vi "UHR-Fleezers Control (host) - 11.9b.vi"() -> ()   [LabVIEW 2014] (continued)
        n1560 = Add(x=w2217, y=w2214) -> (x+y=w2215:i64)
        n1561 = local write "Trap Pos. FB Offset Factor"(w2215) -> ()
        n1562 = xnode "Read/Write Control"("FPGA VI Reference In"=w2221, "error in"=w2220, "Trap Pos. FB Offset Factor"=w2215) -> ()  [unwired: 2 out]
      }
      event "Remove Offset to factor": Value Change {
        n1563 = event-data() -> ()  [unwired: 7 out]
        n1564 = local write "Remove Offset to factor"(FALSE ("Remove Action Offset")) -> ()
        n1565 = local read "Trap Pos. FB Mult Factor"() -> (w2233:i64)
        n1566 = local read "Trap Pos FB Action"() -> (w2231:i64)
        n1567 = local read "Trap Pos. FB Offset Factor"() -> (w2230:i64)
        n1568 = Multiply(x=w2233, y=w2231) -> (x*y=w2232:i64)
        n1569 = local read "Trap Pos. FB Mult Factor"() -> (w2229:i64)
        n1570 = Add(x=w2232, y=w2230) -> (x+y=w2224:i64)
        n1571 = Multiply(x=32768, y="factor") -> (x*y=w2227:dbl)
        n1572 = Multiply(x=w2227, y=w2229) -> (x*y=w2228:dbl)
        n1573 = Subtract(x=w2224, y=w2228) -> (x-y=w2222:dbl)
        n1574 = To Quad Integer(1:w2222) -> (0:w2223:i64)
        n1575 = xnode "Read/Write Control"("FPGA VI Reference In"=w2236, "error in"=w2235, "Trap Pos. FB Offset Factor"=w2223) -> ()  [unwired: 2 out]
        n1576 = local write "Trap Pos. FB Offset Factor"(w2223) -> ()
      }
      event "Trap Pos. FB Range", "Trap Pos. FB Gains", "Trap Pos. FB Mult Factor", "Trap Pos. FB Offset Factor", "Trap Pos FB Negate Action", "Trap Pos FB Monitor\nT1 or T2", "Differential FB?", "Negate Diff?": Value Change {
        n1577 = event-data() -> ()  [unwired: 7 out]
        n1578 = local read "Negate Diff?"() -> (w2237:bool)
        n1579 = xnode "Read/Write Control"("FPGA VI Reference In"=w2247, "error in"=w2246, "Trap Pos. FB Range"="Trap Pos. FB Range", "Trap Pos. FB Gains"="Trap Pos. FB Gains", "Trap Pos. FB Mult Factor"="Trap Pos. FB Mult Factor", "Trap Pos. FB Offset Factor"="Trap Pos. FB Offset Factor", "Trap Pos FB Negate Action"="Trap Pos FB Negate Action", "Trap Pos FB Monitor T1 or T2"="Trap Pos FB Monitor\nT1 or T2", "AI1 X Scale"="Trap Pos. AI1 X Pre-scale", "Negate Diff?"=w2237, "Diff FB Measurement?"="Differential FB?") -> ()  [unwired: 2 out]
      }
      event "Trap Pos FB SP", "Trap Pos FB SP 2", "Use SP 2": Value Change {
        n1580 = event-data() -> ()  [unwired: 7 out]
        n1581 = Select(t="Trap Pos FB SP 2", s="Use SP 2", f="Trap Pos FB SP") -> (s? t:f=w2248:fxp<+/-,16,1>)
        n1582 = xnode "Read/Write Control"("FPGA VI Reference In"=w2253, "error in"=w2252, "Trap Pos. FB SP"=w2248) -> ()  [unwired: 2 out]
      }
      event "Offset SP2 from SP1": Value Change {
        n1583 = event-data() -> ()  [unwired: 7 out]
        n1584 = local read "Trap Pos FB SP"() -> (w2256:fxp<+/-,16,1>)
        n1585 = Add(x=w2256, y="SP2 Offset") -> (x+y=w2254:fxp<+/-,16,1>)
        n1586 = property on="Trap Pos FB SP 2" class="DigNum (strict)"("Val(Sgnl)"=w2254) -> ()  [unwired: 2 in, 2 out]
        n1587 = local write "Offset SP2 from SP1"(FALSE ("Offset SP2 from SP1")) -> ()
      }
      event "Set Reading to\nSetpoint": Value Change {
        # "This is the actual PID input signal"
        n1588 = event-data() -> ()  [unwired: 7 out]
        n1589 = local write "Set Reading to\nSetpoint"(FALSE ("Set SP to Reading")) -> ()
        n1590 = xnode "Read/Write Control"("FPGA VI Reference In"=w2262, "error in"=w2261) -> ("FPGA VI Reference Out"=w2260:T19, "error out"=w2259:errorcluster, "Trap Pos FB Int-Norm Signal"=w2258:fxp<+/-,16,1>)
        n1591 = local read "Differential FB?"() -> (w2263:bool)
        n1592 = case shown="False" w2263 {
          tunnel: [w2268 w2275] -> w2265
          tunnel: w2258 -> [w2266 w2275]
          frame False {
            n1593 = local read "Trap Pos FB Monitor\nT1 or T2"() -> (w2271:bool)
            n1594 = local read "Trap X AI1 (DMA)"() -> (w2274:T13)
            n1595 = Unbundle By Name(w2274) -> ("Set 1"=w2273:fxp<+/-,16,1>, "Set 2"=w2272:fxp<+/-,16,1>)
            n1596 = Select(t=w2273, s=w2271, f=w2272) -> (s? t:f=w2270:fxp<+/-,16,1>)
            n1597 = Not(x="Set SP Using...") -> (.not. x?=w2267:bool)
            n1598 = Select(t=w2266, s=w2267, f=w2270) -> (s? t:f=w2268:fxp<+/-,16,1>)
          }
          frame True {
          }
        }
        n1599 = xnode "Read/Write Control"("FPGA VI Reference In"=w2260, "error in"=w2259, "Trap Pos. FB SP"=w2265) -> ()  [unwired: 2 out]
        n1600 = local write "Trap Pos FB SP"(w2265) -> ()
      }
      event "Trap Pos. FB Out Scale 2^n": Value Change {
        n1601 = event-data() -> ()  [unwired: 7 out]
        n1602 = Scale By Power Of 2(n="Trap Pos. FB Out Scale 2^n", x=ext 1.0) -> (x*2^n=w2276:ext)
        n1603 = property on="Trap Pos. FB Mult Factor" class="DigNum (strict)"("Val(Sgnl)"=w2276) -> ()  [unwired: 2 in, 2 out]
      }
      event "Trap Pos FB Int Count": Value Change {
        n1604 = event-data() -> ()  [unwired: 7 out]
        n1605 = xnode "Read/Write Control"("FPGA VI Reference In"=w2281, "error in"=w2280, "Trap Pos FB Int Count"="Trap Pos FB Int Count") -> ()  [unwired: 2 out]
      }
      event "Trap pos": Value Change {
        n1606 = event-data() -> ()  [unwired: 7 out]
        n1607 = case shown="True" "Trap pos" {
          frame False {
            n1608 = property on="Trap Delta Graph" class="WFGraph (strict)"("Visible"=TRUE) -> ()  [unwired: 2 in, 2 out]
            n1609 = property on="Saved trap pos" class="WFGraph (strict)"("Visible"=FALSE) -> ()  [unwired: 2 in, 2 out]
          }
          frame True {
            n1610 = property on="Saved trap pos" class="WFGraph (strict)"("Visible"=TRUE) -> ()  [unwired: 2 in, 2 out]
            n1611 = property on="Trap Delta Graph" class="WFGraph (strict)"("Visible"=FALSE) -> ()  [unwired: 2 in, 2 out]
          }
        }
      }
      event "Save user params": Value Change {
        n1612 = event-data() -> ()  [unwired: 7 out]
        n1613 = local write "Save user params"(FALSE ("Save user\nparams")) -> ()
        n1614 = call "save control values.vi"("User"="User") -> ()  [unwired: 8 in, 1 out]
        n1615 = local read "Messages"() -> (w2293:string)
        n1616 = Concatenate Strings("User: ", "User", "\r", "Parameters saved.") -> (w2288:string)
        n1617 = call "Update messages.vi"("Message to add"=w2288, "Old message string"=w2293) -> ("New message string"=w2287:string)
        n1618 = local write "Messages"(w2287) -> ()
      }
      event "Load user params": Value Change {
        n1619 = event-data() -> ()  [unwired: 7 out]
        n1620 = local write "Load user params"(FALSE ("Read user\nparams")) -> ()
        n1621 = flat-sequence {
          tunnel: [w2325] -> w2313
          tunnel: [w2324] -> w2311
          tunnel: [w2323] -> w2309
          tunnel: [w2322] -> w2307
          tunnel: [w2321] -> w2305
          tunnel: [w2320] -> w2303
          tunnel: [w2319] -> w2301
          tunnel: [w2318] -> w2299
          tunnel: [w2317] -> w2297
          tunnel: [w2316] -> w2295
          tunnel: [w2335] -> w2314
          tunnel: w2313 -> [w2335]
          tunnel: [w2334] -> w2312
          tunnel: w2311 -> [w2334]
          tunnel: [w2333] -> w2310
          tunnel: w2309 -> [w2333]
          tunnel: [w2332] -> w2308
          tunnel: w2307 -> [w2332]
          tunnel: [w2331] -> w2306
          tunnel: w2305 -> [w2331]
          tunnel: [w2330] -> w2304
          tunnel: w2303 -> [w2330]
          tunnel: [w2329] -> w2302
          tunnel: w2301 -> [w2329]
          tunnel: [w2328] -> w2300
          tunnel: w2299 -> [w2328]
          tunnel: [w2327] -> w2298
          tunnel: w2297 -> [w2327]
          tunnel: [w2326] -> w2296
          tunnel: w2295 -> [w2326]
          tunnel: w2314 -> [w2352]
          tunnel: w2312 -> [w2351]
          tunnel: w2310 -> [w2350]
          tunnel: w2308 -> [w2349]
          tunnel: w2306 -> [w2348]
          tunnel: w2304 -> [w2347]
          tunnel: w2302 -> [w2346]
          tunnel: w2300 -> [w2345]
          tunnel: w2298 -> [w2344]
          tunnel: w2296 -> [w2343]
          frame #0 {
            # "Make exceptions.\nThese will not be\nloaded."
            n1622 = local read "Sample Channel\nFlow"() -> (w2320:bool)
            n1623 = local read "Green ON/Interlacing"() -> (w2321:bool)
            n1624 = local read "Trap 1 (ON/OFF)"() -> (w2325:bool)
            n1625 = local read "Trap 2 (ON/OFF)"() -> (w2324:bool)
            n1626 = local read "Trap Pos. FB ON"() -> (w2316:bool)
            n1627 = local read "Inject Pump 1"() -> (w2319:bool)
            n1628 = local read "Inject Pump 3"() -> (w2318:bool)
            n1629 = local read "Trap D (MHz)"() -> (w2317:dbl)
            n1630 = local read "Index"() -> (w2322:dbl)
            n1631 = local read "Fish"() -> (w2323:bool)
          }
          frame #1 {
            n1632 = local read "User"() -> (w2336:string)
            n1633 = call "retrieve control values.vi"("User"=w2336) -> ()  [unwired: 10 in, 1 out]
            n1634 = local read "Messages"() -> (w2342:string)
            n1635 = Concatenate Strings("User: ", w2336, "\r", "Parameters loaded.") -> (w2337:string)
            n1636 = call "Update messages.vi"("Message to add"=w2337, "Old message string"=w2342) -> ("New message string"=w2341:string)
            n1637 = local write "Messages"(w2341) -> ()
          }
          frame #2 {
            n1638 = local write "Sample Channel\nFlow"(w2347) -> ()
            n1639 = local write "Green ON/Interlacing"(w2348) -> ()
            n1640 = local write "Trap 1 (ON/OFF)"(w2352) -> ()
            n1641 = local write "Trap 2 (ON/OFF)"(w2351) -> ()
            n1642 = local write "Inject Pump 1"(w2346) -> ()
            n1643 = local write "Trap Pos. FB ON"(w2343) -> ()
            n1644 = local write "Inject Pump 3"(w2345) -> ()
            n1645 = local write "Trap D (MHz)"(w2344) -> ()
            n1646 = local write "Index"(w2349) -> ()
            n1647 = local write "Fish"(w2350) -> ()
          }
        }
      }
      event "Abort wiggle": Value Change {
        n1648 = event-data() -> ()  [unwired: 7 out]
        n1649 = flat-sequence {
          tunnel: w2356 -> [w2360]
          tunnel: w2355 -> [w2359]
          tunnel: [w2358] -> w2353
          tunnel: [w2362] -> w2354
          tunnel: w2353 -> [w2362]
          frame #0 {
            n1650 = xnode "Read/Write Control"("FPGA VI Reference In"=w2360, "error in"=w2359, "Abort wiggle 1"="Abort wiggle", "Abort wiggle 2"="Abort wiggle") -> ("error out"=w2358:errorcluster)  [unwired: 1 out]
          }
          frame #1 {
            n1651 = local write "Abort wiggle"(FALSE ("Abort wiggle")) -> ()
          }
        }
      }
    }
    "error out 2" <- w1151
    n1652 = node-c288() -> ()  [unwired: 2 out]
  }
  n1653 = node-c288() -> (w101:T21)  [unwired: 4 in]
  n1654 = local write "Target size"(cluster{"Width":dbl, "Height":dbl} {"Width"=40.0, "Height"=40.0} ("Target size")) -> ()
  n1655 = timed-loop "Run Scripts, including: stage motion" {
    tunnel: w106 -> [w2370]
    tunnel: w105 -> [w2371]
    tunnel: [w2371] -> w104
    tunnel: [w2370] -> w103
    timing: w101 -> [_]
    timing-out: [_] -> w100
    tunnel: w86 -> [w2369]
    tunnel: w87 -> [w2368]
    tunnel: w27 -> [w2365]
    tunnel: w26 -> [w2364]
    tunnel: w25 -> [w2366]
    tunnel: w24 -> [w2367]
    stop <- w2363 stop-if-true
    n1656 = node-c288() -> ()  [unwired: 1 in, 1 out]
    n1657 = event shown="[3] \"Move Cap. 2 (ADig Top)\": Value Change" {
      selector: _ -> [_ _ _ _ _ _ _ _ _ _ _ _ _ _ _ _ _ _ _ _ _]
      dyn-events: _ -> [_ _ _ _ _ _ _ _ _ _ _ _ _ _ _ _ _ _ _ _ _]
      timeout: _ -> [_ _ _ _ _ _ _ _ _ _ _ _ _ _ _ _ _ _ _ _ _]
      tunnel: ["Set Position" "Move to Position" _ _ "Read Harvard" _ _ _ _ _ _ _ "Got ADig bead" "Force FB Script" "Rupture Script" _ "Got DNA bead" "Take Stepping Data" _ "Take Detection Laser\nImage" _] -> _
      tunnel: [_ _ _ _ _ _ _ _ _ _ _ _ _ _ _ _ _ _ _ _ w3043] -> w2363
      tunnel: w2370 -> [w2389 w2397 w2410 w2440 _ w2488 w2528 w2611 w2642 w2776 w2802 w2837 _ w2854 _ _ _ _ _ _ _]
      tunnel: w2371 -> [w2390 w2398 w2411 w2441 _ w2489 w2529 w2612 w2643 w2777 w2803 w2838 _ w2855 _ _ _ _ _ _ _]
      tunnel: w2369 -> [_ _ _ _ w2473 _ _ _ _ _ _ _ _ _ _ _ _ _ _ _ _]
      tunnel: w2368 -> [_ _ _ _ w2472 _ _ _ _ _ _ _ _ _ _ _ _ _ _ _ _]
      tunnel: w2367 -> [_ _ _ _ _ _ _ _ _ _ _ _ _ _ _ _ _ _ _ _ _]
      tunnel: w2366 -> [_ _ _ _ _ _ _ _ _ _ _ _ _ _ _ _ _ _ _ _ _]
      tunnel: w2365 -> [_ _ _ _ _ _ _ _ _ _ _ _ _ _ _ _ _ _ _ _ _]
      tunnel: w2364 -> [_ _ _ _ _ _ _ _ _ _ _ _ _ _ _ _ _ _ _ _ _]
      event "Set Position", "Set Position 2", "Set Position 3", "Set Position 4", "Set Position 5", "Set Position 1": Value Change {
        n1658 = event-data() -> ()  [unwired: 1 in, 5 out]
        n1659 = Build Array("Set Position 1", "Set Position 2", "Set Position 3", "Set Position 4", "Set Position 5") -> (w2388:bool[])
        n1660 = Boolean Array To Number(Boolean array=w2388) -> (number=w2387:u32)
        n1661 = Logarithm Base 2(1:w2387) -> (0:w2379:dbl)
        n1662 = call "Read Stage Position.vi"("error in"=w2389, "VISA resource name in"=w2390) -> ("Current Position"=w2394:cluster{dbl, dbl, dbl}, "error out"=w2393:errorcluster)  [unwired: 2 out]
        n1663 = Decrement(x="Position") -> (x-1=w2377:dbl)
        n1664 = Greater Or Equal?(x=w2379, y=0.0) -> (x >= y?=w2380:bool)
        n1665 = Cluster To Array(cluster=w2394) -> (array=w2391:dbl[])
        n1666 = local write "Stage Control Serial Error"(w2393) -> ()
        n1667 = Select(t=w2379, s=w2380, f=w2377) -> (s? t:f=w2376:dbl)
        n1668 = Increment(x=w2376) -> (x+1=w2375:dbl)
        n1669 = Build Array (concatenate)(w2375, w2391) -> (w2374:dbl[])
        n1670 = Replace Array Subset(array="Saved Stage Positions", new element=w2374, index (row)=w2376) -> (w2392:dbl[][])  [unwired: 1 in]
        n1671 = local write "Saved Stage Positions"(w2392) -> ()
      }
      event "Move to Position": Value Change {
        n1672 = event-data() -> ()  [unwired: 1 in, 5 out]
        n1673 = flat-sequence {
          tunnel: w2398 -> [w2402]
          tunnel: w2397 -> [w2401]
          frame #0 {
            n1674 = local read "Saved Stage Positions"() -> (w2404:dbl[][])
            n1675 = local read "Position"() -> (w2403:dbl)
            n1676 = local write "Stage Moving"(TRUE ("Stage Moving")) -> ()
            n1677 = call "move to saved stage position.vi"("error in"=w2401, "Stage VISA resource name in"=w2402, "Position"=w2403, "Saved Stage Positions"=w2404) -> ("error out"=w2400:errorcluster)  [unwired: 1 out]
            n1678 = local write "Stage Control Serial Error"(w2400) -> ()
          }
          frame #1 {
            n1679 = call <vilib>:"Beep.vi"() -> ()  [unwired: 3 in, 9 out]
            n1680 = local write "Stage Moving"(FALSE ("Stage Moving")) -> ()
          }
        }
      }
      event "Move Cap. 1 (DNA Bottom)": Value Change {
        n1681 = event-data() -> ()  [unwired: 1 in, 5 out]
        n1682 = local write "Move Cap. 1 (DNA Bottom)"(FALSE ("Move Cap. 1 (DNA Right)")) -> ()
        n1683 = flat-sequence {
          tunnel: w2410 -> [w2413]
          tunnel: w2411 -> [w2414]
          tunnel: [w2414] -> w2408
          tunnel: [w2413] -> w2407
          tunnel: w2408 -> [w2416]
          tunnel: w2407 -> [w2415]
          frame #0 {
            n1684 = property on="Sample Channel\nFlow" class="Bool (strict)"("Val(Sgnl)"="Cap 1 Samp Flow ON") -> ()  [unwired: 2 in, 2 out]
          }
          frame #1 {
            n1685 = local read "Saved Stage Positions"() -> (w2426:dbl[][])
            n1686 = local write "Stage Moving"(TRUE ("Stage Moving")) -> ()
            n1687 = Array Subset(array=w2426, index (row)=0 ("index"), length (row)=1 ("length"), index (col)=1 ("index"), length (col)=3 ("length")) -> (w2423:dbl[][])
            n1688 = Reshape Array(w2423, 3 ("dimension size")) -> (w2421:dbl[])
            n1689 = Array To Cluster(array=w2421) -> (cluster=w2420:cluster{"[0]":dbl, "[1]":dbl, "[2]":dbl})
            n1690 = call "Set Stage Position.vi"("Position"=w2420, "error in"=w2415, "VISA resource name in"=w2416) -> ("error out"=w2419:errorcluster)  [unwired: 2 out]
            n1691 = local write "Stage Control Serial Error"(w2419) -> ()
          }
          frame #2 {
            n1692 = local write "Stage Moving"(FALSE ("Stage Moving")) -> ()
            n1693 = case shown="True" "Cap 1 Flow ON" {
              frame False {
              }
              frame True {
                n1694 = property on="Inject Pump 1" class="Bool (strict)"("Val(Sgnl)"=TRUE ("Value (Signaling)")) -> ()  [unwired: 2 in, 2 out]
              }
            }
            n1695 = call <vilib>:"Beep.vi"() -> ()  [unwired: 3 in, 9 out]
          }
          frame #3 {
            n1696 = property on="Sample Channel\nFlow" class="Bool (strict)"("Val(Sgnl)"=FALSE ("Value (Signaling)")) -> ()  [unwired: 2 in, 2 out]
            n1697 = local read "Cap. 2 BD T1?\n(ADig T1, DNA T2)"() -> (w2433:bool)
            n1698 = case shown="True" w2433 {
              tunnel: "Cap 1 T ON" -> [w2435 w2436]
              frame False {
                n1699 = property on="Trap 1 (ON/OFF)" class="Bool (strict)"("Val(Sgnl)"=w2435) -> ()  [unwired: 2 in, 2 out]
              }
              frame True {
                n1700 = property on="Trap 2 (ON/OFF)" class="Bool (strict)"("Val(Sgnl)"=w2436) -> ()  [unwired: 2 in, 2 out]
              }
            }
            n1701 = property on="Got DNA bead" class="Bool"("Key Focus"=TRUE) -> ()  [unwired: 2 in, 2 out]
          }
        }
      }
      event "Move Cap. 2 (ADig Top)": Value Change {
        n1702 = event-data() -> ()  [unwired: 1 in, 5 out]
        n1703 = local write "Move Cap. 2 (ADig Top)"(FALSE ("Move Cap. 2 (ADig Left)")) -> ()
        n1704 = flat-sequence {
          tunnel: w2440 -> [w2443]
          tunnel: w2441 -> [w2444]
          tunnel: [w2444] -> w2438
          tunnel: [w2443] -> w2437
          tunnel: w2438 -> [w2446]
          tunnel: w2437 -> [w2445]
          frame #0 {
            n1705 = property on="Sample Channel\nFlow" class="Bool (strict)"("Val(Sgnl)"="Cap 2 Samp Flow ON") -> ()  [unwired: 2 in, 2 out]
          }
          frame #1 {
            n1706 = local read "Saved Stage Positions"() -> (w2456:dbl[][])
            n1707 = local write "Stage Moving"(TRUE ("Stage Moving")) -> ()
            n1708 = Array Subset(array=w2456, index (row)=1 ("index"), length (row)=1 ("length"), index (col)=1 ("index"), length (col)=3 ("length")) -> (w2453:dbl[][])
            n1709 = disable-structure shown="Disabled" {
              frame Disabled {
                w2458 = FALSE ("Value (Signaling)")
                n1710 = property on="Trap 1 (ON/OFF)" class="Bool (strict)"("Val(Sgnl)"=w2458) -> ()  [unwired: 2 in, 2 out]
                n1711 = property on="Trap 1 (ON/OFF)" class="Bool (strict)"("Val(Sgnl)"=w2458) -> ()  [unwired: 2 in, 2 out]
              }
              frame Enabled {
              }
            }
            n1712 = Reshape Array(w2453, 3 ("dimension size")) -> (w2451:dbl[])
            n1713 = Array To Cluster(array=w2451) -> (cluster=w2450:cluster{"[0]":dbl, "[1]":dbl, "[2]":dbl})
            n1714 = call "Set Stage Position.vi"("Position"=w2450, "error in"=w2445, "VISA resource name in"=w2446) -> ("error out"=w2449:errorcluster)  [unwired: 2 out]
            n1715 = local write "Stage Control Serial Error"(w2449) -> ()
          }
          frame #2 {
            n1716 = local write "Stage Moving"(FALSE ("Stage Moving")) -> ()
            n1717 = call <vilib>:"Beep.vi"() -> ()  [unwired: 3 in, 9 out]
            n1718 = case shown="True" "Cap 2 Flow ON" {
              frame False {
              }
              frame True {
                n1719 = property on="Inject Pump 3" class="Bool (strict)"("Val(Sgnl)"=TRUE ("Value (Signaling)")) -> ()  [unwired: 2 in, 2 out]
              }
            }
          }
          frame #3 {
            n1720 = Wait (ms)(milliseconds to wait=u32 500) -> ()  [unwired: 1 out]
          }
          frame #4 {
            n1721 = local read "Cal @ (MHz)"() -> (w2464:dbl)
            n1722 = property on="Sample Channel\nFlow" class="Bool (strict)"("Val(Sgnl)"=FALSE ("Value (Signaling)")) -> ()  [unwired: 2 in, 2 out]
            n1723 = case shown="False" "Cap. 2 BD T1?\n(ADig T1, DNA T2)" {
              tunnel: "Cap 2 T ON" -> [w2469 w2470]
              frame False {
                n1724 = property on="Trap 2 (ON/OFF)" class="Bool (strict)"("Val(Sgnl)"=w2469) -> ()  [unwired: 2 in, 2 out]
              }
              frame True {
                n1725 = property on="Trap 1 (ON/OFF)" class="Bool (strict)"("Val(Sgnl)"=w2470) -> ()  [unwired: 2 in, 2 out]
              }
            }
            n1726 = property on="Got ADig bead" class="Bool"("Key Focus"=TRUE) -> ()  [unwired: 2 in, 2 out]
            n1727 = local write "Target"("Target\nON?") -> ()
            n1728 = property on="Trap D (MHz)" class="DigNum (strict)"("Val(Sgnl)"=w2464) -> ()  [unwired: 2 in, 2 out]
          }
        }
      }
      event "Read Harvard": Value Change {
        n1729 = event-data() -> ()  [unwired: 1 in, 5 out]
        n1730 = Concatenate Strings("write buffer", "\r") -> (w2475:string)
        n1731 = VISA Write(VISA resource name=w2473, write buffer=w2475, error in (no error)=w2472) -> (VISA resource name out=w2484:refnum<visa-resource-name>, error out=w2483:errorcluster)  [unwired: 1 out]
        n1732 = stacked-sequence {
          tunnel: [w2487] -> w2482
          tunnel: w2484 -> [w2487]
          tunnel: w2483 -> [w2486]
          tunnel: [w2486] -> w2477
          frame #0 {
            n1733 = Wait (ms)(milliseconds to wait=50) -> ()  [unwired: 1 out]
          }
        }
        n1734 = property class="Instr"(reference=w2482, error in=w2477) -> (reference out=w2481:refnum<visa-resource-name>, error out=w2479:errorcluster, "Serial Settings:Number of Bytes at Serial Port"=w2480:u32)
        "Serial Settings:Number of Bytes at Serial Port" <- w2480
        n1735 = VISA Read(VISA resource name=w2481, byte count=w2480, error in (no error)=w2479) -> (read buffer=w2478:string)  [unwired: 3 out]
        "read buffer" <- w2478
        n1736 = Fract/Exp String To Number(string=w2478) -> ()  [unwired: 5 out]
      }
      event "+z", "-z": Value Change {
        n1737 = event-data() -> ()  [unwired: 1 in, 5 out]
        n1738 = flat-sequence {
          tunnel: w2488 -> [w2510]
          tunnel: w2489 -> [w2490]
          frame #0 {
            n1739 = call "Read Stage Position.vi"("error in"=w2510, "VISA resource name in"=w2490) -> ("Current Position"=w2495:cluster{dbl, dbl, dbl}, "error out"=w2508:errorcluster, "VISA resource name out"=w2509:refnum<visa-resource-name>)  [unwired: 1 out]
            n1740 = local read "Saved Stage Positions"() -> (w2519:dbl[][])
            n1741 = Divide(x="z nudge increment (um)", y=1000.0) -> (x/y=w2507:dbl)
            n1742 = Boolean To (0,1)(Boolean="+z") -> (0, 1=w2499:i16)
            n1743 = Boolean To (0,1)(Boolean="-z") -> (0, 1=w2500:i16)
            n1744 = Array Subset(array=w2519, index (row)=1 ("index"), length (row)=1 ("length"), index (col)=1 ("index"), length (col)=3 ("length")) -> (w2516:dbl[][])
            n1745 = Multiply(x=w2499, y=w2507) -> (x*y=w2503:dbl)
            n1746 = Multiply(x=w2500, y=w2507) -> (x*y=w2501:dbl)
            n1747 = Unbundle(w2495) -> (w2493:dbl, w2492:dbl, w2496:dbl)
            n1748 = Negate(x=w2501) -> (-x=w2502:dbl)
            n1749 = Reshape Array(w2516, 3 ("dimension size")) -> (w2514:dbl[])
            n1750 = Add(x=w2503, y=w2502) -> (x+y=w2504:dbl)
            n1751 = Array To Cluster(array=w2514) -> ()  [unwired: 1 out]
            n1752 = Add(x=w2504, y=w2496) -> (x+y=w2494:dbl)
            n1753 = Bundle(cluster=w2495, w2493, w2492, w2494) -> (w2491:cluster{dbl, dbl, dbl})
            n1754 = call "Set Stage Position.vi"("Position"=w2491, "error in"=w2508, "VISA resource name in"=w2509) -> ("error out"=w2513:errorcluster)  [unwired: 2 out]
            n1755 = local write "Stage Moving"(TRUE ("Stage Moving")) -> ()
            n1756 = local write "Stage Control Serial Error"(w2513) -> ()
          }
          frame #1 {
            n1757 = local write "Stage Moving"(FALSE ("Stage Moving")) -> ()
            n1758 = call <vilib>:"Beep.vi"() -> ()  [unwired: 3 in, 9 out]
          }
        }
      }
      event "Cal/Data Acq. Spot": Value Change {
        n1759 = event-data() -> ()  [unwired: 1 in, 5 out]
        n1760 = flat-sequence {
          tunnel: w2528 -> [w2532]
          tunnel: w2529 -> [w2533]
          tunnel: [w2533] -> w2525
          tunnel: [w2532] -> w2524
          tunnel: w2525 -> [w2538]
          tunnel: w2524 -> [w2537]
          tunnel: ["Cal @ (MHz)"] -> w2522
          tunnel: [w2542] -> w2526
          tunnel: w2522 -> [w2542]
          tunnel: w2526 -> [w2553]
          tunnel: ["W/ Offset 1"] -> w2523
          tunnel: w2526 -> [w2574]
          tunnel: w2523 -> [w2572]
          frame #0 {
            n1761 = property on="Sample Channel\nFlow" class="Bool (strict)"("Val(Sgnl)"="Daq spot flow on") -> ()  [unwired: 2 in, 2 out]
            n1762 = Wait (ms)(milliseconds to wait=u32 250) -> ()  [unwired: 1 out]
          }
          frame #1 {
            n1763 = local read "Saved Stage Positions"() -> (w2535:dbl[][])
            n1764 = property on="Trap D (MHz)" class="DigNum (strict)"("Val(Sgnl)"="Cal @ (MHz)") -> ()  [unwired: 2 in, 2 out]
            n1765 = local write "Stage Moving"(TRUE ("Stage Moving")) -> ()
            n1766 = call "move to saved stage position.vi"("error in"=w2537, "Stage VISA resource name in"=w2538, "Position"="Cal Stage Position", "Saved Stage Positions"=w2535) -> ("error out"=w2536:errorcluster)  [unwired: 1 out]
            n1767 = local write "Stage Control Serial Error"(w2536) -> ()
          }
          frame #2 {
            n1768 = local write "Stage Moving"(FALSE ("Stage Moving")) -> ()
            n1769 = property on="Sample Channel\nFlow" class="Bool (strict)"("Val(Sgnl)"="Flow ON\nduring cal?") -> ()  [unwired: 2 in, 2 out]
            n1770 = call <vilib>:"Beep.vi"() -> ()  [unwired: 3 in, 9 out]
          }
          frame #3 {
            n1771 = local read "Wait Before Save (s)"() -> (w2545:u32)
            n1772 = Multiply(x=w2545, y=u32 1000 ("milliseconds to wait")) -> (x*y=w2546:u32)
            n1773 = Wait (ms)(milliseconds to wait=w2546) -> ()  [unwired: 1 out]
          }
          frame #4 {
            n1774 = property on="Save Calibration" class="Bool (strict)"("Val(Sgnl)"=TRUE ("Value (Signaling)")) -> ()  [unwired: 2 in, 2 out]
          }
          frame #5 {
            n1775 = Wait (ms)(milliseconds to wait=u32 2000) -> ()  [unwired: 1 out]
          }
          frame #6 {
            # "Check to see if \nsaving done"
            n1776 = while {
              stop <- w2549 stop-if-true
              n1777 = local read "Saving..."() -> (w2550:bool)
              n1778 = Wait (ms)(milliseconds to wait=u32 100) -> ()  [unwired: 1 out]
              n1779 = Not(x=w2550) -> (.not. x?=w2549:bool)
            }
          }
          frame #7 {
            n1780 = case shown="True" "W/ Offset 1" {
              tunnel: w2553 -> [_ w2554]
              frame False {
              }
              frame True {
                n1781 = stacked-sequence {
                  tunnel: w2554 -> [_ _ _ _ _ _ _ w2571]
                  frame #0 {
                    n1782 = property on="Trap D (MHz)" class="DigNum (strict)"("Val(Sgnl)"="Offset 1 Start (MHz)") -> ()  [unwired: 2 in, 2 out]
                    n1783 = Replace Array Subset(array=u32[] [0] ("Index Values"), new element="Offset 1 Set", index=0) -> (w2555:u32[])
                    n1784 = property on="Saved AOD Raster Scan Parameter Sets" class="Arr (strict)"("Index Values"=w2555) -> ()  [unwired: 2 in, 2 out]
                  }
                  frame #1 {
                    n1785 = Wait (ms)(milliseconds to wait=u32 200) -> ()  [unwired: 1 out]
                  }
                  frame #2 {
                    n1786 = property on="Load parameters" class="Bool (strict)"("Val(Sgnl)"=TRUE ("Value (Signaling)")) -> ()  [unwired: 2 in, 2 out]
                  }
                  frame #3 {
                    n1787 = Wait (ms)(milliseconds to wait=u32 200) -> ()  [unwired: 1 out]
                  }
                  frame #4 {
                    n1788 = property on="Trap Raster Scan" class="Bool (strict)"("Val(Sgnl)"=TRUE ("Value (Signaling)")) -> ()  [unwired: 2 in, 2 out]
                  }
                  frame #5 {
                    n1789 = Wait (ms)(milliseconds to wait=u32 2000) -> ()  [unwired: 1 out]
                  }
                  frame #6 {
                    n1790 = while {
                      stop <- w2568 stop-if-true
                      n1791 = local read "Raster Scanning..."() -> (w2570:bool)
                      n1792 = local read "Saving..."() -> (w2566:bool)
                      n1793 = Wait (ms)(milliseconds to wait=u32 100) -> ()  [unwired: 1 out]
                      n1794 = Not(x=w2566) -> (.not. x?=w2565:bool)
                      n1795 = Not(x=w2570) -> (.not. x?=w2567:bool)
                      n1796 = And(x=w2567, y=w2565) -> (x .and. y?=w2568:bool)
                    }
                  }
                  frame #7 {
                    n1797 = property on="Trap D (MHz)" class="DigNum (strict)"("Val(Sgnl)"=w2571) -> ()  [unwired: 2 in, 2 out]
                  }
                }
              }
            }
          }
          frame #8 {
            n1798 = local read "Save ave N"() -> (w2573:dbl)
            n1799 = case shown="False" "W/ Offset 2" {
              tunnel: w2574 -> [_ w2581]
              tunnel: w2573 -> [_ w2580]
              tunnel: w2572 -> [w2576 _]
              frame False {
                n1800 = case shown="False" w2576 {
                  frame False {
                    n1801 = Multiply(x="Cal read wait (s)", y=u32 1000 ("milliseconds to wait")) -> (x*y=w2578:u32)
                    n1802 = Wait (ms)(milliseconds to wait=w2578) -> ()  [unwired: 1 out]
                  }
                  frame True {
                  }
                }
              }
              frame True {
                n1803 = stacked-sequence {
                  tunnel: w2581 -> [_ _ _ _ _ _ _ _ _ w2602 _ _]
                  tunnel: w2580 -> [_ _ _ _ _ _ _ _ _ w2600 _ _]
                  frame #0 {
                    n1804 = property on="Save ave N" class="DigNum (strict)"("Val(Sgnl)"=1.0 ("Value (Signaling)")) -> ()  [unwired: 2 in, 2 out]
                  }
                  frame #1 {
                    n1805 = Wait (ms)(milliseconds to wait=u32 500) -> ()  [unwired: 1 out]
                  }
                  frame #2 {
                    n1806 = property on="Trap D (MHz)" class="DigNum (strict)"("Val(Sgnl)"="Offset 2 Start (MHz)") -> ()  [unwired: 2 in, 2 out]
                    n1807 = Replace Array Subset(array=u32[] [0] ("Index Values"), new element="Offset 2 Set", index=0) -> (w2586:u32[])
                    n1808 = property on="Saved AOD Raster Scan Parameter Sets" class="Arr (strict)"("Index Values"=w2586) -> ()  [unwired: 2 in, 2 out]
                  }
                  frame #3 {
                    n1809 = Wait (ms)(milliseconds to wait=u32 500) -> ()  [unwired: 1 out]
                  }
                  frame #4 {
                    n1810 = property on="Load parameters" class="Bool (strict)"("Val(Sgnl)"=TRUE ("Value (Signaling)")) -> ()  [unwired: 2 in, 2 out]
                  }
                  frame #5 {
                    n1811 = Wait (ms)(milliseconds to wait=u32 500) -> ()  [unwired: 1 out]
                  }
                  frame #6 {
                    n1812 = property on="Trap Raster Scan" class="Bool (strict)"("Val(Sgnl)"=TRUE ("Value (Signaling)")) -> ()  [unwired: 2 in, 2 out]
                  }
                  frame #7 {
                    n1813 = Wait (ms)(milliseconds to wait=u32 2000) -> ()  [unwired: 1 out]
                  }
                  frame #8 {
                    n1814 = while {
                      stop <- w2595 stop-if-true
                      n1815 = local read "Raster Scanning..."() -> (w2598:bool)
                      n1816 = local read "Saving..."() -> (w2596:bool)
                      n1817 = Wait (ms)(milliseconds to wait=u32 100) -> ()  [unwired: 1 out]
                      n1818 = Not(x=w2596) -> (.not. x?=w2594:bool)
                      n1819 = Not(x=w2598) -> (.not. x?=w2597:bool)
                      n1820 = And(x=w2597, y=w2594) -> (x .and. y?=w2595:bool)
                    }
                  }
                  frame #9 {
                    n1821 = property on="Trap D (MHz)" class="DigNum (strict)"("Val(Sgnl)"=w2602) -> ()  [unwired: 2 in, 2 out]
                    n1822 = property on="Saved AOD Raster Scan Parameter Sets" class="Arr (strict)"("Index Values"=u32[] [0]) -> ()  [unwired: 2 in, 2 out]
                    n1823 = property on="Save ave N" class="DigNum (strict)"("Val(Sgnl)"=w2600) -> ()  [unwired: 2 in, 2 out]
                  }
                  frame #10 {
                    n1824 = Wait (ms)(milliseconds to wait=u32 500) -> ()  [unwired: 1 out]
                  }
                  frame #11 {
                    n1825 = property on="Load parameters" class="Bool (strict)"("Val(Sgnl)"=TRUE ("Value (Signaling)")) -> ()  [unwired: 2 in, 2 out]
                  }
                }
              }
            }
          }
          frame #9 {
            n1826 = property on="Read Cal" class="Bool (strict)"("Val(Sgnl)"=TRUE ("Value (Signaling)")) -> ()  [unwired: 2 in, 2 out]
          }
          frame #10 {
            n1827 = Wait (ms)(milliseconds to wait=u32 1000) -> ()  [unwired: 1 out]
          }
          frame #11 {
            n1828 = property on="Fish" class="Bool (strict)"("Val(Sgnl)"=TRUE ("Value (Signaling)")) -> ()  [unwired: 2 in, 2 out]
          }
        }
        n1829 = local write "Cal/Data Acq. Spot"(FALSE ("Cal/Data Acq. Spot")) -> ()
      }
      event "Dump Beads": Value Change {
        n1830 = event-data() -> ()  [unwired: 1 in, 5 out]
        n1831 = flat-sequence {
          tunnel: ["Dump spot flow on?"] -> w2608
          tunnel: [w2620] -> w2609
          tunnel: w2608 -> [w2620]
          tunnel: w2612 -> [w2625]
          tunnel: w2611 -> [w2624]
          tunnel: [w2622] -> w2610
          tunnel: w2609 -> [w2622]
          tunnel: w2610 -> [w2636]
          frame #0 {
            w2613 = FALSE ("Value (Signaling)")
            n1832 = local read "Saving..."() -> (w2615:bool)
            n1833 = local write "Dump Beads"(FALSE ("Dump Beads")) -> ()
            n1834 = property on="Inject Pump 3" class="Bool (strict)"("Val(Sgnl)"=w2613) -> ()  [unwired: 2 in, 2 out]
            n1835 = property on="Inject Pump 1" class="Bool (strict)"("Val(Sgnl)"=w2613) -> ()  [unwired: 2 in, 2 out]
            n1836 = local write "Stop Saving"(w2615) -> ()
            n1837 = local write "Fish"(w2613) -> ()
          }
          frame #1 {
            w2616 = TRUE
            w2617 = FALSE ("Fl. Triggered...")
            n1838 = case shown="True" "Dump spot flow on?" {
              frame False {
              }
              frame True {
                n1839 = property on="Sample Channel\nFlow" class="Bool (strict)"("Val(Sgnl)"=TRUE ("Stage Moving")) -> ()  [unwired: 2 in, 2 out]
              }
            }
            n1840 = local write "Fl. Triggered..."(w2617) -> ()
            n1841 = local write "Tether"(w2617) -> ()
            n1842 = local write "Multiple tether"(w2617) -> ()
            n1843 = local write "Good tether"(w2617) -> ()
            n1844 = property on="Green ON/Interlacing" class="Bool (strict)"("Val(Sgnl)"=w2617) -> ()  [unwired: 2 in, 2 out]
            n1845 = property on="Trap Pos. FB ON" class="Bool (strict)"("Val(Sgnl)"=w2617) -> ()  [unwired: 2 in, 2 out]
            n1846 = property on="Trap Trig. Fl." class="Bool (strict)"("Val(Sgnl)"=w2617) -> ()  [unwired: 2 in, 2 out]
            n1847 = local write "Bad fit"(w2617) -> ()
            n1848 = local write "Hysteresis"(w2617) -> ()
            n1849 = property on="Fl. Triggered..." class="Bool (strict)"("Val(Sgnl)"=w2617) -> ()  [unwired: 2 in, 2 out]
            n1850 = local write "Restart DMA? (AOD)"(w2616) -> ()
            n1851 = local write "Save scans"(w2616) -> ()
            n1852 = property on="Dip for Protein" class="Bool (strict)"("Val(Sgnl)"=w2617) -> ()  [unwired: 2 in, 2 out]
            n1853 = property on="Pause dwell" class="Bool (strict)"("Val(Sgnl)"=w2617) -> ()  [unwired: 2 in, 2 out]
          }
          frame #2 {
            n1854 = property on="Trap Pos. FB Offset Factor" class="DigNum (strict)"("Val(Sgnl)"=i64 0 ("Value (Signaling)")) -> ()  [unwired: 2 in, 2 out]
          }
          frame #3 {
            n1855 = local read "Saved Stage Positions"() -> (w2626:dbl[][])
            n1856 = Array Subset(array=w2626, index (row)=3 ("index"), length (row)=1 ("length"), index (col)=1 ("index"), length (col)=3 ("length")) -> (w2631:dbl[][])
            n1857 = local write "Stage Moving"(TRUE ("Stage Moving")) -> ()
            n1858 = Reshape Array(w2631, 3 ("dimension size")) -> (w2629:dbl[])
            n1859 = Array To Cluster(array=w2629) -> (cluster=w2628:cluster{"[0]":dbl, "[1]":dbl, "[2]":dbl})
            n1860 = call "Set Stage Position.vi"("Position"=w2628, "error in"=w2624, "VISA resource name in"=w2625) -> ()  [unwired: 3 out]
          }
          frame #4 {
            w2637 = FALSE ("Value (Signaling)")
            n1861 = case shown="True" w2636 {
              frame False {
              }
              frame True {
                n1862 = property on="Sample Channel\nFlow" class="Bool (strict)"("Val(Sgnl)"=FALSE ("Stage Moving")) -> ()  [unwired: 2 in, 2 out]
              }
            }
            n1863 = property on="Trap 1 (ON/OFF)" class="Bool (strict)"("Val(Sgnl)"=w2637) -> ()  [unwired: 2 in, 2 out]
            n1864 = property on="Trap 2 (ON/OFF)" class="Bool (strict)"("Val(Sgnl)"=w2637) -> ()  [unwired: 2 in, 2 out]
            n1865 = call <vilib>:"Beep.vi"() -> ()  [unwired: 3 in, 9 out]
            n1866 = local write "Fish"(FALSE ("Fish for Tether")) -> ()
          }
          frame #5 {
            n1867 = property on="Move Cap. 2 (ADig Top)" class="Bool (strict)"("Val(Sgnl)"=TRUE ("Value (Signaling)")) -> ()  [unwired: 2 in, 2 out]
            n1868 = property on="Tab Control" class="TabCtl (strict)"("Val(Sgnl)"=T4."Status" ("Value (Signaling)")) -> ()  [unwired: 2 in, 2 out]
          }
        }
      }
      event "Dip for Protein": Value Change {
        n1869 = event-data() -> ()  [unwired: 1 in, 5 out]
        n1870 = case shown="True" "Dip for Protein" {
          tunnel: w2643 -> [_ w2645]
          tunnel: w2642 -> [_ w2644]
          frame False {
          }
          frame True {
            n1871 = while {
              tunnel: w2645 -> [w2656]
              tunnel: w2644 -> [w2655]
              i -> [w2651]
              stop <- w2646 stop-if-true
              n1872 = Increment(x=w2651) -> (x+1=→"Dip #":i32)
              n1873 = flat-sequence {
                tunnel: w2655 -> [w2667]
                tunnel: w2656 -> [w2668]
                tunnel: [w2668] -> w2660
                tunnel: [w2667] -> w2659
                tunnel: [w2661] -> w2647
                tunnel: [w2673] -> w2654
                tunnel: [w2674] -> w2653
                tunnel: w2660 -> [w2675]
                tunnel: w2659 -> [w2676]
                tunnel: [w2671] -> w2648
                tunnel: w2647 -> [w2671]
                tunnel: [w2684] -> w2658
                tunnel: w2654 -> [w2684]
                tunnel: [w2683] -> w2657
                tunnel: w2653 -> [w2683]
                tunnel: [w2680] -> w2652
                tunnel: [w2679] -> w2649
                tunnel: w2648 -> [w2679]
                tunnel: w2657 -> [w2704]
                tunnel: w2658 -> [w2705]
                tunnel: w2652 -> [w2706]
                tunnel: w2649 -> [w2703]
                tunnel: [w2765] -> w2646
                frame #0 {
                  n1874 = local read "Trap Pos. FB ON"() -> (w2661:bool)
                  n1875 = Compound Arithmetic op=AND("Flow ON\nduring dip?", "FB OFF when \nflow ON", w2661) -> (w2662:bool)
                  n1876 = case shown="True" "Move trap \nbefore dip move?" {
                    frame False {
                    }
                    frame True {
                      n1877 = property on="Trap D (MHz)" class="DigNum (strict)"("Val(Sgnl)"="Dipping D (MHz)") -> ()  [unwired: 2 in, 2 out]
                    }
                  }
                  n1878 = property on="Green ON/Interlacing" class="Bool (strict)"("Val(Sgnl)"="Green ON\nbefore dip?") -> ()  [unwired: 2 in, 2 out]
                  n1879 = property on="Sample Channel\nFlow" class="Bool (strict)"("Val(Sgnl)"="Flow ON\nduring dip?") -> ()  [unwired: 2 in, 2 out]
                  n1880 = case shown="True" w2662 {
                    frame False {
                    }
                    frame True {
                      n1881 = property on="Trap Pos. FB ON" class="Bool (strict)"("Val(Sgnl)"=FALSE ("Value (Signaling)")) -> ()  [unwired: 2 in, 2 out]
                    }
                  }
                }
                frame #1 {
                  n1882 = local read "Saved Stage Positions"() -> (w2678:dbl[][])
                  n1883 = local write "Cancel dwell"(FALSE ("Cancel dwell")) -> ()
                  n1884 = call "move to saved stage position.vi"("error in"=w2676, "Stage VISA resource name in"=w2675, "Position"="Dip Stage \nPosition", "Saved Stage Positions"=w2678) -> ("VISA resource name out"=w2673:refnum<visa-resource-name>, "error out"=w2674:errorcluster)
                }
                frame #2 {
                  n1885 = node-c288() -> (w2682:T21)  [unwired: 4 in]
                  n1886 = timed-loop {
                    timing: w2682 -> [_]
                    timing-out: [_] -> w2681
                    tunnel: [w2688] -> w2680
                    i -> [w2685]
                    stop <- w2689 stop-if-true
                    n1887 = node-c288() -> ()  [unwired: 1 in, 1 out]
                    n1888 = Greater Or Equal?(x=w2685, y="Dip Duration (s)") -> (x >= y?=w2697:bool)
                    n1889 = local read "Dip for Protein"() -> (w2690:bool)
                    n1890 = local read "Dump Beads"() -> (w2687:bool)
                    n1891 = local read "Cancel dwell"() -> (w2696:bool)
                    n1892 = local read "Pause dwell"() -> (w2693:bool)
                    n1893 = Not(x=w2690) -> (.not. x?=w2695:bool)
                    n1894 = Compound Arithmetic op=OR(w2696, w2697, w2695) -> (w2694:bool)
                    n1895 = Select(t=FALSE, s=w2693, f=w2694) -> (s? t:f=w2691:bool)
                    n1896 = Not(x=w2687) -> (.not. x?=w2686:bool)
                    n1897 = node-c288() -> ()  [unwired: 1 in, 1 out]
                    n1898 = And(x=w2690, y=w2686) -> (x .and. y?=w2688:bool)
                    n1899 = Or(x=w2691, y=w2687) -> (x .or. y?=w2689:bool)
                    "Dip Time (s)" <- w2685
                  }
                  n1900 = node-c288(w2681) -> ()  [unwired: 1 out]
                }
                frame #3 {
                  n1901 = case shown="True" w2706 {
                    tunnel: w2705 -> [_ w2711]
                    tunnel: w2704 -> [_ w2710]
                    tunnel: w2703 -> [_ w2707]
                    frame False {
                    }
                    frame True {
                      n1902 = flat-sequence {
                        tunnel: w2710 -> [w2715]
                        tunnel: w2711 -> [w2716]
                        tunnel: [w2716] -> w2709
                        tunnel: [w2715] -> w2708
                        tunnel: w2707 -> [w2712]
                        tunnel: w2709 -> [w2726]
                        tunnel: w2708 -> [w2725]
                        tunnel: w2707 -> [w2734]
                        frame #0 {
                          n1903 = local read "Sample Channel\nFlow"() -> (w2714:bool)
                          n1904 = case shown="True" w2714 {
                            tunnel: "Flow ON \nduring return\nfrom dip?" -> [w2717 w2720]
                            tunnel: w2712 -> [_ w2719]
                            frame False {
                              n1905 = case shown="True" w2717 {
                                frame False {
                                }
                                frame True {
                                n1906 = property on="Sample Channel\nFlow" class="Bool (strict)"("Val(Sgnl)"=TRUE ("Value (Signaling)")) -> ()  [unwired: 2 in, 2 out]
                                }
                              }
                            }
                            frame True {
                              n1907 = case shown="False" w2720 {
                                tunnel: w2719 -> [w2721 _]
                                frame False {
                                n1908 = property on="Trap Pos. FB ON" class="Bool (strict)"("Val(Sgnl)"=w2721) -> ()  [unwired: 2 in, 2 out]
                                n1909 = property on="Sample Channel\nFlow" class="Bool (strict)"("Val(Sgnl)"=FALSE ("Value (Signaling)")) -> ()  [unwired: 2 in, 2 out]
                                }
                                frame True {
                                }
                              }
                            }
                          }
                        }
                        frame #1 {
                          # "For turning on green laser before stage reaches lower spot"
                          n1910 = case shown="True" "Green ON\nafter start\nreturn?" {
                            frame False {
                            }
                            frame True {
                              n1911 = flat-sequence {
                                frame #0 {
                                n1912 = Multiply(x="Green delay after \nstart return (s)", y=1000.0) -> (x*y=w2731:dbl)
                                n1913 = Wait (ms)(milliseconds to wait=w2731) -> ()  [unwired: 1 out]
                                }
                                frame #1 {
                                n1914 = property on="Green ON/Interlacing" class="Bool (strict)"("Val(Sgnl)"=TRUE ("Value (Signaling)")) -> ()  [unwired: 2 in, 2 out]
                                }
                              }
                            }
                          }
                          n1915 = local read "Saved Stage Positions"() -> (w2729:dbl[][])
                          n1916 = local write "Cancel dwell"(FALSE ("Cancel dwell")) -> ()
                          n1917 = call "move to saved stage position.vi"("error in"=w2725, "Stage VISA resource name in"=w2726, "Position"="Return Stage \nPosition", "Saved Stage Positions"=w2729) -> ("error out"=w2727:errorcluster)  [unwired: 1 out]
                          n1918 = local write "Stage Control Serial Error"(w2727) -> ()
                        }
                        frame #2 {
                          n1919 = property on="Trap Pos. FB ON" class="Bool (strict)"("Val(Sgnl)"=w2734) -> ()  [unwired: 2 in, 2 out]
                          n1920 = case shown="True" "Green ON \nafter return?" {
                            frame False {
                            }
                            frame True {
                              n1921 = property on="Green ON/Interlacing" class="Bool (strict)"("Val(Sgnl)"=TRUE ("Value (Signaling)")) -> ()  [unwired: 2 in, 2 out]
                            }
                          }
                          n1922 = case shown="True" "Move trap after return?" {
                            frame False {
                            }
                            frame True {
                              n1923 = property on="Trap D (MHz)" class="DigNum (strict)"("Val(Sgnl)"="Dip Trap D 2 (MHz)") -> ()  [unwired: 2 in, 2 out]
                            }
                          }
                          n1924 = case shown="True" "Save data after return?" {
                            frame False {
                            }
                            frame True {
                              n1925 = property on="Start Saving" class="Bool (strict)"("Val(Sgnl)"=TRUE ("Value (Signaling)")) -> ()  [unwired: 2 in, 2 out]
                            }
                          }
                          n1926 = property on="Sample Channel\nFlow" class="Bool (strict)"("Val(Sgnl)"="Flow ON\nduring daq?") -> ()  [unwired: 2 in, 2 out]
                        }
                        frame #3 {
                          n1927 = node-c288() -> (w2743:T21)  [unwired: 4 in]
                          n1928 = timed-loop {
                            timing: w2743 -> [_]
                            timing-out: [_] -> w2742
                            i -> [w2744]
                            stop <- w2746 stop-if-true
                            n1929 = node-c288() -> ()  [unwired: 1 in, 1 out]
                            n1930 = local read "Dump Beads"() -> (w2745:bool)
                            n1931 = Greater Or Equal?(x=w2744, y="Dwell Duration (s)") -> (x >= y?=w2751:bool)
                            n1932 = local read "Dip for Protein"() -> (w2748:bool)
                            n1933 = Not(x=w2748) -> (.not. x?=w2747:bool)
                            n1934 = Compound Arithmetic op=OR(w2751, "Cancel dwell", w2747) -> (w2750:bool)
                            n1935 = node-c288() -> ()  [unwired: 1 in, 1 out]
                            n1936 = Select(t=FALSE, s="Pause dwell", f=w2750) -> (s? t:f=w2753:bool)
                            n1937 = Or(x=w2753, y=w2745) -> (x .or. y?=w2746:bool)
                            "Dwell Time (s)" <- w2744
                          }
                          n1938 = node-c288(w2742) -> ()  [unwired: 1 out]
                        }
                      }
                    }
                  }
                }
                frame #4 {
                  n1939 = local read "Dip for Protein"() -> (w2762:bool)
                  n1940 = local read "Tether"() -> (w2761:bool)
                  n1941 = local read "Dump Beads"() -> (w2763:bool)
                  n1942 = local write "Cancel dwell"(FALSE ("Cancel dwell")) -> ()
                  n1943 = Not(x=w2761) -> (.not. x?=w2760:bool)
                  n1944 = Not(x=w2762) -> (.not. x?=w2766:bool)
                  n1945 = Not(x="Cont. Repeat Dipping?") -> (.not. x?=w2768:bool)
                  n1946 = Compound Arithmetic op=OR(w2760, w2766, w2768, w2763) -> (w2765:bool)
                }
              }
            }
          }
        }
      }
      event "Profile": Value Change {
        n1947 = event-data() -> ()  [unwired: 1 in, 5 out]
        n1948 = flat-sequence {
          tunnel: w2777 -> [w2780]
          tunnel: w2776 -> [w2788]
          tunnel: [w2782] -> w2775
          tunnel: [w2781] -> w2774
          tunnel: [w2779] -> w2772
          tunnel: [w2778] -> w2769
          tunnel: w2775 -> [w2795]
          tunnel: w2774 -> [w2794]
          tunnel: [w2792] -> w2773
          tunnel: w2772 -> [w2793]
          tunnel: [w2791] -> w2771
          tunnel: [w2790] -> w2770
          tunnel: w2769 -> [w2790]
          tunnel: w2773 -> [w2799]
          tunnel: w2771 -> [w2798]
          tunnel: w2770 -> [w2797]
          frame #0 {
            n1949 = call "Read Stage Position.vi"("error in"=w2788, "VISA resource name in"=w2780) -> ("Current Position"=w2778:cluster{dbl, dbl, dbl}, "error out"=w2781:errorcluster, "VISA resource name out"=w2779:refnum<visa-resource-name>)  [unwired: 1 out]
            "Current Position" <- w2778
            n1950 = local write "Stage Control Serial Error"(w2781) -> ()
            n1951 = Unbundle(w2778) -> (w2785:dbl, w2787:dbl, w2783:dbl)
            n1952 = Add(x=w2787, y="Y change (mm)") -> (x+y=w2784:dbl)
            n1953 = Bundle(w2785, w2784, w2783) -> (w2782:cluster{dbl, dbl, dbl})  [unwired: 1 in]
          }
          frame #1 {
            # "move to new position and start saving"
            n1954 = local write "Stage Moving"(TRUE ("Stage Moving")) -> ()
            n1955 = local write "Start Saving"(TRUE ("Start Saving")) -> ()
            n1956 = call "Set Stage Position.vi"("Position"=w2795, "error in"=w2794, "VISA resource name in"=w2793) -> ("error out"=w2791:errorcluster, "VISA resource name out"=w2792:refnum<visa-resource-name>)  [unwired: 1 out]
          }
          frame #2 {
            # "go back to start"
            n1957 = call "Set Stage Position.vi"("Position"=w2797, "error in"=w2798, "VISA resource name in"=w2799) -> ()  [unwired: 3 out]
          }
          frame #3 {
            # "stop saving"
            n1958 = local write "Stop Saving"(TRUE ("Stop Saving")) -> ()
            n1959 = local write "Stage Moving"(FALSE ("Stage Moving")) -> ()
          }
        }
      }
      event "Move to Position 1", "Move to Position 2", "Move to Position 3", "Move to Position 4", "Move to Position 5", "Lower Ch. Cap.": Value Change {
        n1960 = event-data() -> ()  [unwired: 1 in, 5 out]
